vi "temp.vi"() -> ()   [LabVIEW 2020]
panel:
  out "Temperature Chart":dbl(graph)
  out "TEMPERARUE":dbl
  out "Meter":dbl(knob) scale=0.0..30.0
  out "HIGH":bool
  out "MEDIUM":bool
  out "LOW":bool
  in  "Slide":dbl(slide) caption="C" scale=0.0..30.0
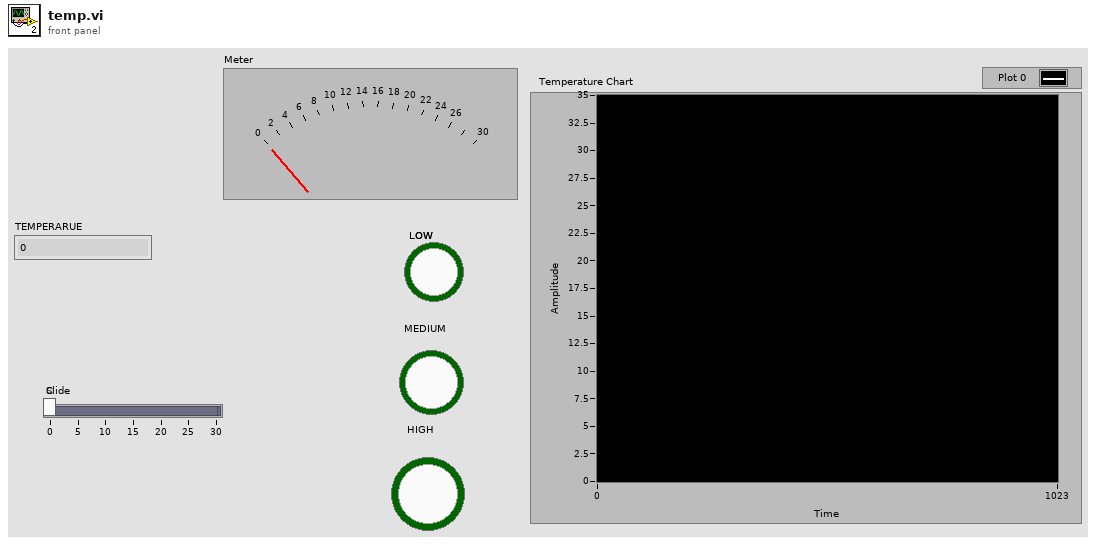
[diagram p1: front panel]
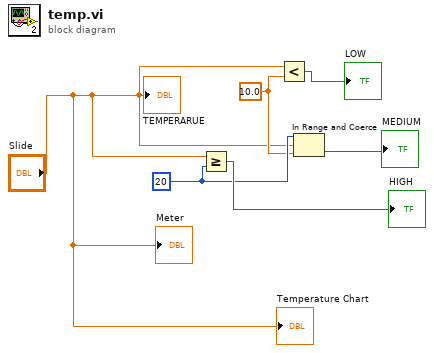
[diagram p0: block diagram]
diagram:
  w3 = 10.0 ("x")
  w4 = 20
  n1 = Greater Or Equal?(x="Slide", y=w4) -> (x >= y?=→"HIGH":bool)
  n2 = Less?(x="Slide", y=w3) -> (x < y?=→"LOW":bool)
  n3 = In Range and Coerce(upper limit=w4, x="Slide", lower limit=w3) -> (In Range?=→"MEDIUM":bool)  [unwired: 1 out]
  "Meter" <- "Slide"
  "TEMPERARUE" <- "Slide"
  "Temperature Chart" <- "Slide"
